vi "臂环接收机.vi"() -> ()   [LabVIEW 2023]
uses:
  <vilib>/Instr/_visa.llb/VISA Flush IO Buffer Mask.ctl
  <vilib>/Instr/_visa.llb/VISA Configure Serial Port (Instr).vi
panel:
  out "chn1":i32(graph)
  out "gry":cluster{i16, i16, i16}(graph)
  out "acc":cluster{i16, i16, i16}(graph)
  out "chn6":i32(graph)
  out "chn5":i32(graph)
  out "chn2":i32(graph)
  out "chn8":i32(graph)
  out "chn4":i32(graph)
  out "chn7":i32(graph)
  out "chn3":i32(graph)
  in  "write_buffer":string
  in  "发送按钮":bool
  out "ReadBuffer":string
  out "读取返回数":u32
  in  "serial":refnum<visa-resource-name> caption="VISA资源名称"
  in  "串口开关":bool
  out "串口状态":bool
  # "念通智能臂环软件——测试阶段试用版本"
  # "臂环通道1波形"
  # "臂环通道5波形"
  # "臂环通道2波形"
  # "臂环通道6波形"
  # "臂环通道3波形"
  # "臂环通道7波形"
  # "臂环通道4波形"
  # "臂环通道8波形"
  # "臂环角速度"
  # "臂环加速度表"
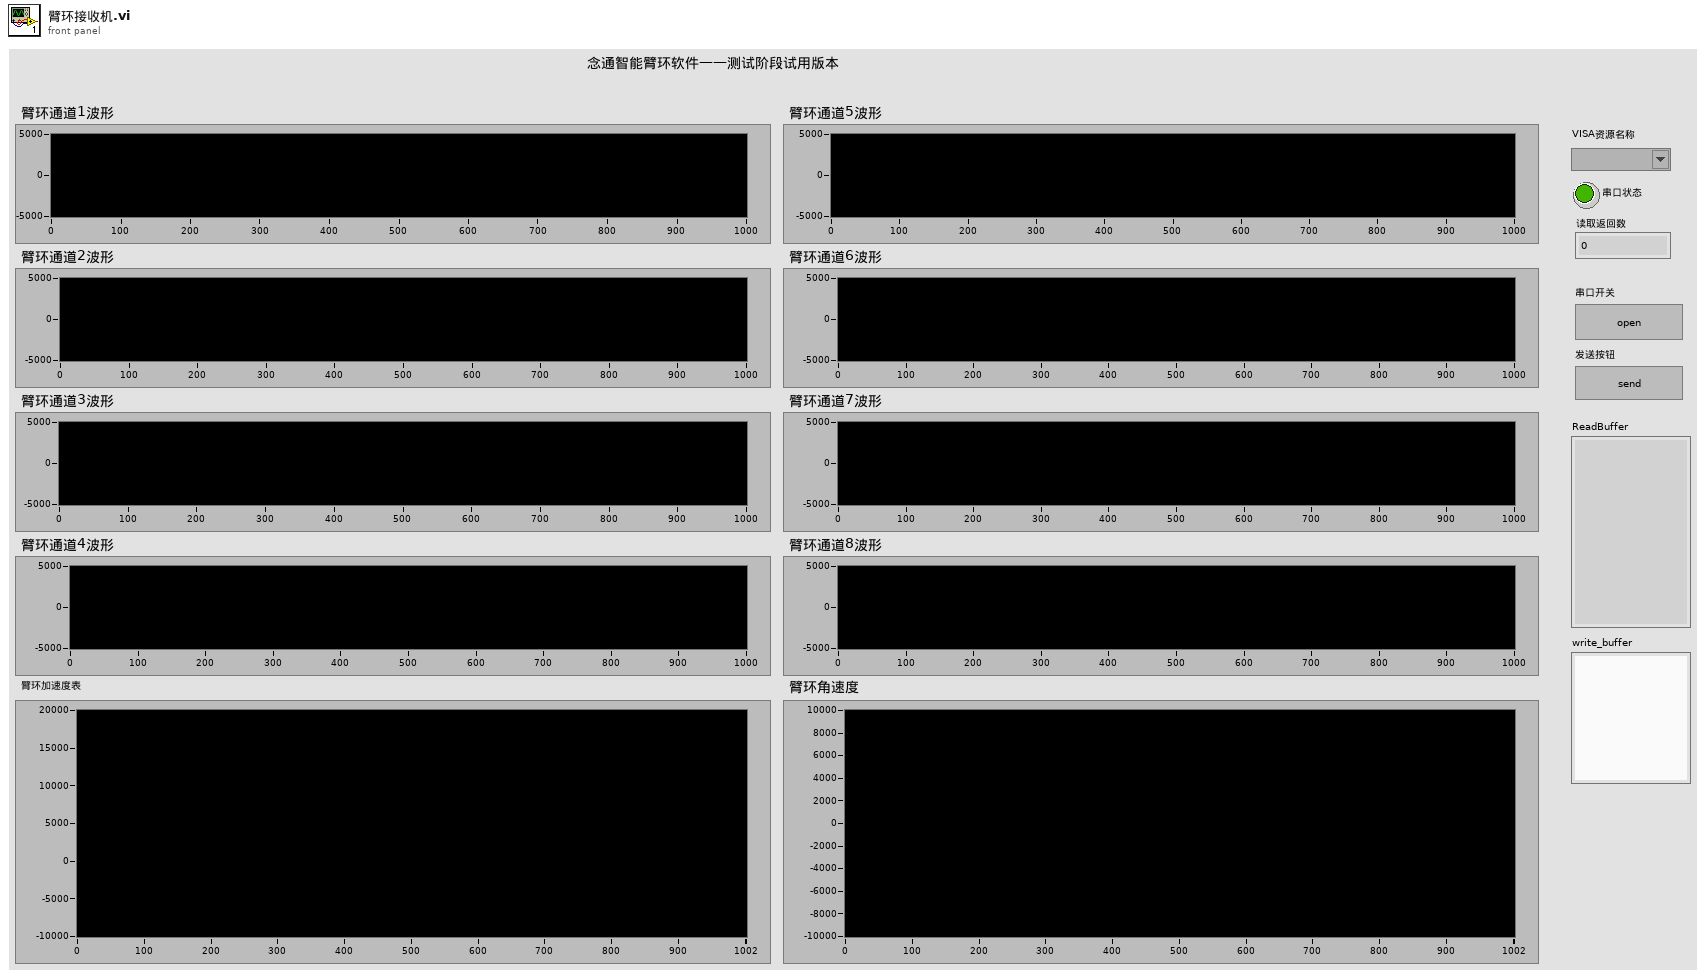
[diagram p1: front panel]
types:
  T1 = enum16{"nohead", "get_bb", "get_aa", "none_4bytes", "get_crc", "get_bat", "get_cnt"}
  T2 = cluster{"rx_cnt":u32, "rx_finish":bool, "head":enum16{"nohead", "get_bb", "get_aa", "none_4bytes", "get_crc", "get_bat", "get_cnt"}, "rx_len":u32, "data_len":u32, "crc":u8, "bat_lev":u8, "data":u8[], "none_4byte":u8[], "rx_4byte_len":u8}
  T3 = typedef "状态机控件.ctl" = enum16{"init_state", "main_state", "uart_receive_state", "stop_state"}
  T4 = typedef "VISA Flush IO Buffer Mask.ctl" = u16
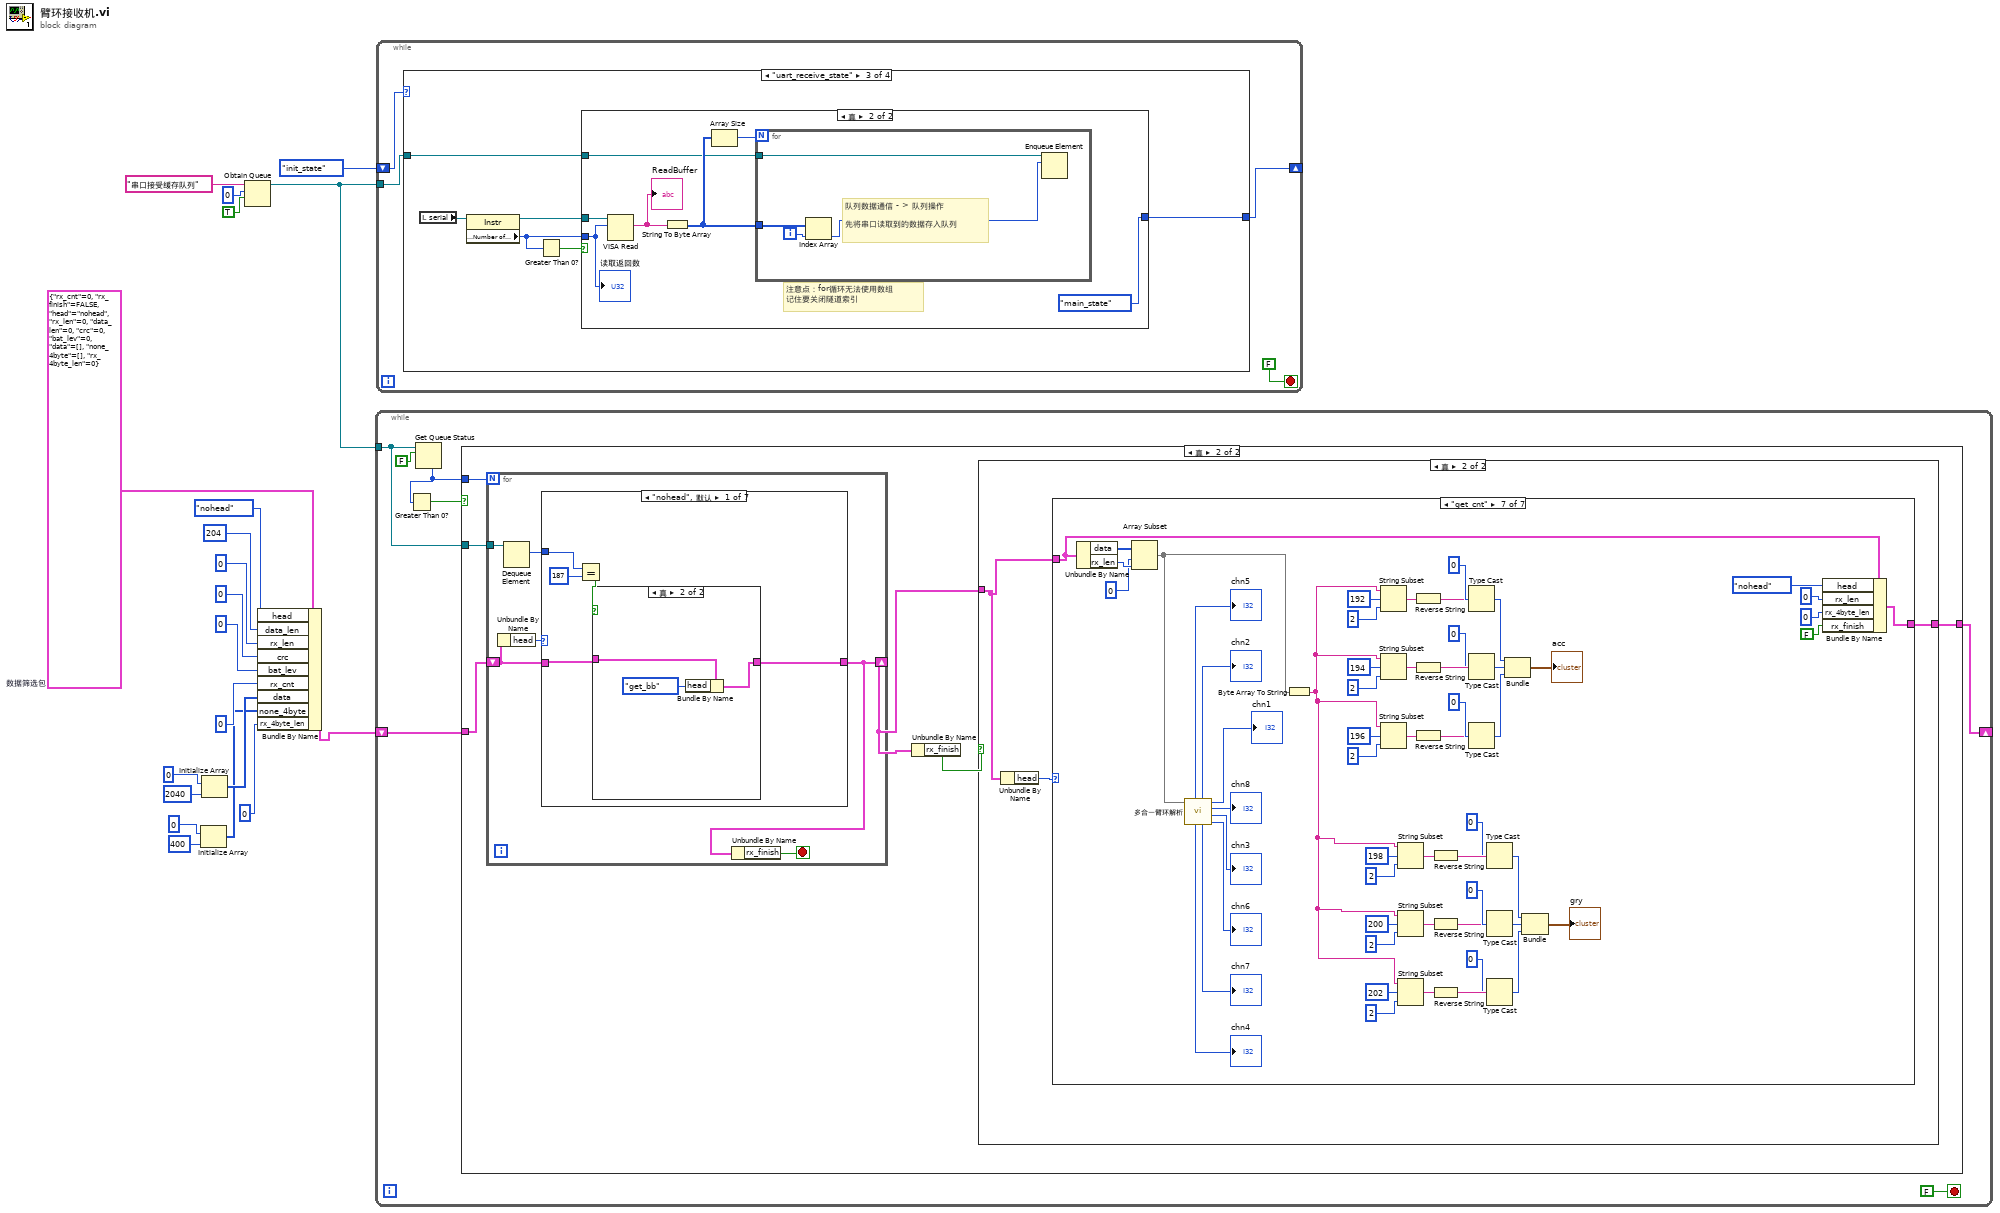
[diagram p0: block diagram]
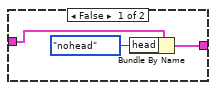
[diagram p10: hidden frame]
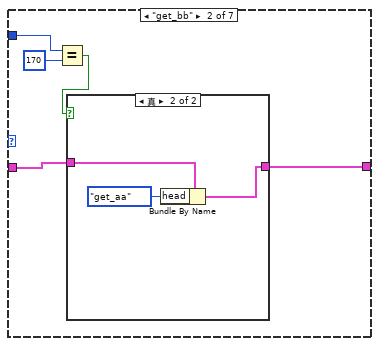
[diagram p11: hidden frame]
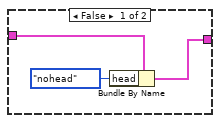
[diagram p12: hidden frame]
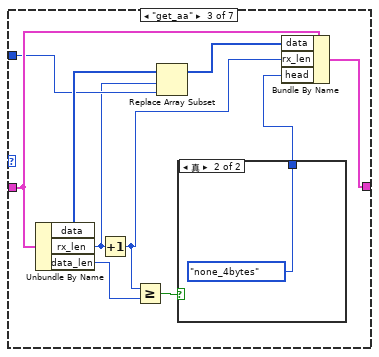
[diagram p13: hidden frame]
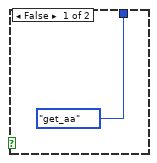
[diagram p14: hidden frame]
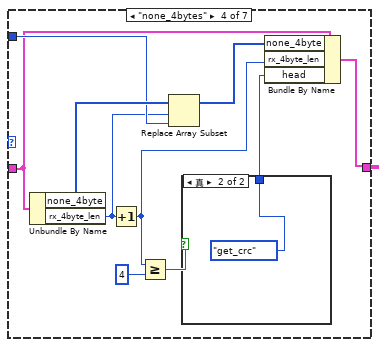
[diagram p15: hidden frame]
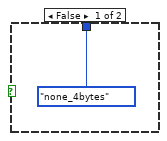
[diagram p16: hidden frame]
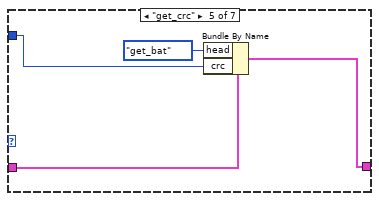
[diagram p17: hidden frame]
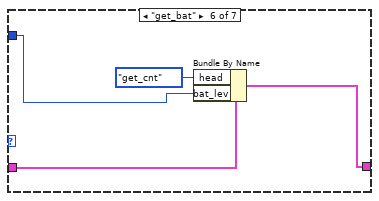
[diagram p18: hidden frame]
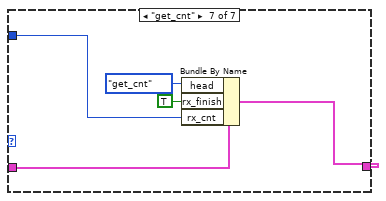
[diagram p19: hidden frame]
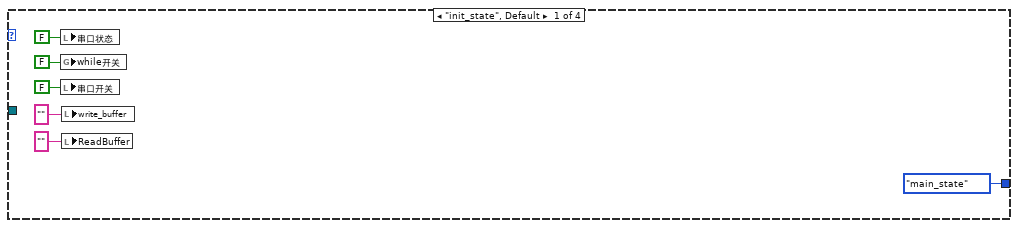
[diagram p20: hidden frame]
diagram:
  w2 = T2 {"rx_cnt"=0, "rx_finish"=FALSE, "head"=enum."nohead", "rx_len"=0, "data_len"=0, "crc"=0, "bat_lev"=0, "data"=[], "none_4byte"=[], "rx_4byte_len"=0}  # 数据筛选包
  n1 = Initialize Array(u8 0 ("元素"), 400 ("维数大小")) -> (w5:u8[])
  n2 = Initialize Array(u8 0 ("元素"), 2040 ("维数大小")) -> (w10:u8[])
  n3 = Obtain Queue(name (unnamed)="串口接受缓存队列" ("名称（未命名）"), element data type=u8 0, create if not found? (T)=TRUE ("如未找到则创建？(T)")) -> (queue out=w16:refnum<queue>)  [unwired: 2 in, 2 out]
  n4 = Bundle By Name(cluster=w2, "head"=T1."nohead", "data_len"=204, "rx_len"=0, "crc"=0, "bat_lev"=0, "rx_cnt"=u32 0, "data"=w10, "none_4byte"=w5, "rx_4byte_len"=u8 0) -> (w1:T2)
  n5 = while {
    tunnel: w16 -> [w22]
    shift-right: [w21] -> _
    shift-left: w1 -> [w23]
    stop <- FALSE stop-if-true
    n6 = Get Queue Status(queue=w22, return elements? (F)=FALSE ("返回元素？(F)")) -> (# elements in queue=w24:i32)  [unwired: 1 in, 7 out]
    n7 = Greater Than 0?(x=w24) -> (x > 0?=w25:bool)
    n8 = case shown="真" w25 {
      tunnel: w24 -> [_ w34]
      tunnel: w23 -> [w28 w33]
      tunnel: w22 -> [_ w32]
      tunnel: [w28 w29] -> w21
      frame False {
      }
      frame True {
        n9 = for {
          N: w34 -> [_]
          tunnel: w32 -> [w107]
          shift-right: [w103] -> w30
          shift-left: w33 -> [w104]
          stop <- w102 stop-if-true
          n10 = Unbundle By Name(w104) -> ("head"=w106:T1)
          n11 = Dequeue Element(queue=w107) -> (element=w105:u8)  [unwired: 2 in, 3 out]
          n12 = case shown="\"nohead\", 默认" w106 {
            tunnel: w105 -> [w111 w122 w135 w148 w155 w159 w165]
            tunnel: w104 -> [w109 w120 w139 w146 w157 w161 w166]
            tunnel: [w108 w119 w130 w142 w154 w158 w162] -> w103
            frame "nohead", Default {
              n13 = Equal?(x=w111, y=u8 187) -> (x = y?=w110:bool)
              n14 = case shown="真" w110 {
                tunnel: w109 -> [w115 w118]
                tunnel: [w113 w117] -> w108
                frame False {
                  n15 = Bundle By Name(cluster=w115, "head"=T1."nohead") -> (w113:T2)
                }
                frame True {
                  n16 = Bundle By Name(cluster=w118, "head"=T1."get_bb") -> (w117:T2)
                }
              }
            }
            frame "get_bb" {
              n17 = Equal?(x=w122, y=u8 170) -> (x = y?=w121:bool)
              n18 = case shown="真" w121 {
                tunnel: w120 -> [w125 w128]
                tunnel: [w124 w127] -> w119
                frame False {
                  n19 = Bundle By Name(cluster=w125, "head"=T1."nohead") -> (w124:T2)
                }
                frame True {
                  n20 = Bundle By Name(cluster=w128, "head"=T1."get_aa") -> (w127:T2)
                }
              }
            }
            frame "get_aa" {
              n21 = Unbundle By Name(w139) -> ("data"=w136:u8[], "rx_len"=w134:u32, "data_len"=w138:u32)
              n22 = Increment(x=w134) -> (x+1=w133:u32)
              n23 = Greater Or Equal?(x=w133, y=w138) -> (x >= y?=w137:bool)
              n24 = Replace Array Subset(array=w136, new element=w135, index=w134) -> (w132:u8[])
              n25 = case shown="真" w137 {
                tunnel: [T1."get_aa" ("head") T1."none_4bytes" ("head")] -> w131
                frame False {
                }
                frame True {
                }
              }
              n26 = Bundle By Name(cluster=w139, "data"=w132, "rx_len"=w133, "head"=w131) -> (w130:T2)
            }
            frame "none_4bytes" {
              n27 = Unbundle By Name(w146) -> ("none_4byte"=w149:u8[], "rx_4byte_len"=w147:u8)
              n28 = Increment(x=w147) -> (x+1=w144:u8)
              n29 = Greater Or Equal?(x=w144, y=u8 4) -> (x >= y?=w151:bool)
              n30 = Replace Array Subset(array=w149, new element=w148, index=w147) -> (w145:u8[])
              n31 = case shown="真" w151 {
                tunnel: [T1."none_4bytes" ("head") T1."get_crc" ("head")] -> w143
                frame False {
                }
                frame True {
                }
              }
              n32 = Bundle By Name(cluster=w146, "none_4byte"=w145, "rx_4byte_len"=w144, "head"=w143) -> (w142:T2)
            }
            frame "get_crc" {
              n33 = Bundle By Name(cluster=w157, "head"=T1."get_bat", "crc"=w155) -> (w154:T2)
            }
            frame "get_bat" {
              n34 = Bundle By Name(cluster=w161, "head"=T1."get_cnt", "bat_lev"=w159) -> (w158:T2)
            }
            frame "get_cnt" {
              n35 = Bundle By Name(cluster=w166, "head"=T1."get_cnt", "rx_finish"=TRUE, "rx_cnt"=w165) -> (w162:T2)
            }
          }
          n36 = Unbundle By Name(w103) -> ("rx_finish"=w102:bool)
        }
        n37 = Unbundle By Name(w30) -> ("rx_finish"=w31:bool)
        n38 = case shown="真" w31 {
          tunnel: w30 -> [w35 w37]
          tunnel: [w35 w36] -> w29
          frame False {
          }
          frame True {
            n39 = Unbundle By Name(w37) -> ("head"=w38:T1)
            n40 = case shown="\"get_cnt\"" w38 {
              tunnel: w37 -> [w39 w40 w41 w42 w43 w44 w98]
              tunnel: [w39 w40 w41 w42 w43 w44 w93] -> w36
              frame "nohead", Default {
              }
              frame "get_bb" {
              }
              frame "get_aa" {
              }
              frame "none_4bytes" {
              }
              frame "get_crc" {
              }
              frame "get_bat" {
              }
              frame "get_cnt" {
                n41 = Unbundle By Name(w98) -> ("data"=w101:u8[], "rx_len"=w100:u32)
                n42 = Array Subset(array=w101, index=u32 0 ("索引"), length=w100) -> (w85:u8[])
                n43 = call "多合一臂环解析.vi"("数组"=w85) -> ("chn6"=→"chn6":i32, "chn3"=→"chn3":i32, "chn8"=→"chn8":i32, "chn1"=→"chn1":i32, "chn7"=→"chn7":i32, "chn2"=→"chn2":i32, "chn4"=→"chn4":i32, "chn5"=→"chn5":i32)  [unwired: 3 in]
                n44 = Byte Array To String(unsigned byte array=w85) -> (string=w46:string)
                n45 = String Subset(string=w46, offset (0)=192 ("偏移量(0)"), length (rest)=2 ("长度（剩余）")) -> (substring=w82:string)
                n46 = String Subset(string=w46, offset (0)=194 ("偏移量(0)"), length (rest)=2 ("长度（剩余）")) -> (substring=w76:string)
                n47 = String Subset(string=w46, offset (0)=196 ("偏移量(0)"), length (rest)=2 ("长度（剩余）")) -> (substring=w71:string)
                n48 = String Subset(string=w46, offset (0)=198 ("偏移量(0)"), length (rest)=2 ("长度（剩余）")) -> (substring=w49:string)
                n49 = String Subset(string=w46, offset (0)=200 ("偏移量(0)"), length (rest)=2 ("长度（剩余）")) -> (substring=w55:string)
                n50 = String Subset(string=w46, offset (0)=202 ("偏移量(0)"), length (rest)=2 ("长度（剩余）")) -> (substring=w60:string)
                n51 = Reverse String(1:w82) -> (0:w80:string)
                n52 = Reverse String(1:w76) -> (0:w78:string)
                n53 = Reverse String(1:w71) -> (0:w69:string)
                n54 = Reverse String(1:w49) -> (0:w51:string)
                n55 = Reverse String(1:w55) -> (0:w53:string)
                n56 = Reverse String(1:w60) -> (0:w62:string)
                n57 = Type Cast(type=i16 0, x=w80) -> (*(type *) &x=w79:i16)
                n58 = Type Cast(type=i16 0, x=w78) -> (*(type *) &x=w68:i16)
                n59 = Type Cast(type=i16 0, x=w69) -> (*(type *) &x=w67:i16)
                n60 = Type Cast(type=i16 0, x=w51) -> (*(type *) &x=w52:i16)
                n61 = Type Cast(type=i16 0, x=w53) -> (*(type *) &x=w63:i16)
                n62 = Type Cast(type=i16 0, x=w62) -> (*(type *) &x=w64:i16)
                n63 = Bundle(w79, w68, w67) -> (→"acc":cluster{i16, i16, i16})  [unwired: 1 in]
                n64 = Bundle(w52, w63, w64) -> (→"gry":cluster{i16, i16, i16})  [unwired: 1 in]
                n65 = Bundle By Name(cluster=w98, "head"=T1."nohead", "rx_len"=u8 0, "rx_4byte_len"=u8 0, "rx_finish"=FALSE) -> (w93:T2)
              }
            }
          }
        }
      }
    }
  }
  n66 = while {
    shift-right: [w170] -> _
    shift-left: 状态机控件."init_state" ("枚举") -> [w169]
    tunnel: w16 -> [w168]
    stop <- FALSE stop-if-true
    n67 = case shown="\"uart_receive_state\"" w169 {
      tunnel: [状态机控件."main_state" ("枚举") w178 w213 状态机控件."stop_state" ("枚举")] -> w170
      tunnel: w168 -> [_ _ w208 _]
      frame "init_state", Default {
        n68 = local write "串口状态"(FALSE ("串口状态")) -> ()
        n69 = global write "枚举全局变量.vi" "while开关"(FALSE ("全局变量while开关")) -> ()
        n70 = local write "串口开关"(FALSE ("串口状态")) -> ()
        n71 = local write "write_buffer"("" ("write_buffer")) -> ()
        n72 = local write "ReadBuffer"("" ("ReadBuffer")) -> ()
      }
      frame "main_state" {
        n73 = event shown="[1] \"串口开关\": 值改变" {
          selector: _ -> [_ _ _]
          dyn-events: _ -> [_ _ _]
          timeout: 0 -> [_ _ _]
          tunnel: [w180 w183 w201] -> w178
          event Timeout {
            n74 = event-data() -> ()  [unwired: 1 in, 3 out]
            n75 = local read "串口状态"() -> (w179:bool)
            n76 = case shown="假" w179 {
              tunnel: [状态机控件."main_state" ("枚举") 状态机控件."uart_receive_state" ("枚举")] -> w180
              frame False {
              }
              frame True {
              }
            }
          }
          event "串口开关": Value Change {
            n77 = event-data() -> ()  [unwired: 1 in, 6 out]
            n78 = case shown="假" "串口开关" {
              tunnel: [状态机控件."main_state" ("枚举") w188] -> w183
              frame False {
                # "关闭串口"
                n79 = local read "serial"() -> (w186:refnum<visa-resource-name>)
                n80 = local write "串口状态"(FALSE ("串口状态")) -> ()
                n81 = VISA Close(VISA resource name=w186) -> ()  [unwired: 1 in, 1 out]
              }
              frame True {
                n82 = call-poly "VISA Configure Serial Port"("VISA resource name"="serial", "baud rate (9600)"=u32 921600) -> ("error out"=w191:errorcluster)  [unwired: 12 in, 1 out]
                n83 = Unbundle By Name(w191) -> ("status"=w190:bool)
                n84 = Not(x=w190) -> (.not. x?=w189:bool)
                "串口状态" <- w189
                n85 = case shown="真" w189 {
                  tunnel: [状态机控件."main_state" ("枚举") 状态机控件."uart_receive_state" ("枚举")] -> w188
                  frame False {
                    n86 = local write "串口开关"(FALSE ("串口状态")) -> ()
                    n87 = One Button Dialog(message="串口打开失败" ("消息")) -> ()  [unwired: 1 in, 1 out]
                  }
                  frame True {
                    w197 = T4 16 items=["清空接收缓冲区"=16, "向设备写入传输缓冲区"=32, "清空接收缓冲区（无I/O）"=64, "清空传输缓冲区"=128] ("Mask")
                    n88 = local read "serial"() -> (w198:refnum<visa-resource-name>)
                    n89 = VISA Flush I/O Buffer(VISA resource name=w198, mask (16)=w197) -> ()  [unwired: 1 in, 2 out]
                  }
                }
              }
            }
          }
          event "发送按钮": Value Change {
            n90 = event-data() -> ()  [unwired: 1 in, 6 out]
            n91 = local read "串口状态"() -> (w200:bool)
            n92 = case shown="真" w200 {
              tunnel: [状态机控件."main_state" ("枚举") 状态机控件."uart_receive_state" ("枚举")] -> w201
              frame False {
                n93 = One Button Dialog(message="打开串口后在发送" ("消息")) -> ()  [unwired: 1 in, 1 out]
              }
              frame True {
                n94 = global write "枚举全局变量.vi" "while开关"(FALSE ("while开关")) -> ()
                n95 = local read "serial"() -> (w207:refnum<visa-resource-name>)
                n96 = VISA Write(VISA resource name=w207, write buffer="write_buffer") -> ()  [unwired: 1 in, 3 out]
              }
            }
          }
        }
      }
      frame "uart_receive_state" {
        n97 = local read "serial"() -> (w209:refnum<visa-resource-name>)
        n98 = property class="Instr"(reference=w209) -> (reference out=w211:refnum<visa-resource-name>, "Serial Settings:Number of Bytes at Serial Port"=w210:u32)  [unwired: 1 in, 1 out]
        n99 = Greater Than 0?(x=w210) -> (x > 0?=w212:bool)
        n100 = case shown="真" w212 {
          tunnel: [状态机控件."main_state" ("枚举") 状态机控件."main_state" ("枚举")] -> w213
          tunnel: w211 -> [_ w220]
          tunnel: w210 -> [_ w219]
          tunnel: w208 -> [_ w215]
          frame False {
          }
          frame True {
            # "注意点：for循环无法使用数组\n记住要关闭隧道索引"
            n101 = VISA Read(VISA resource name=w220, byte count=w219) -> (read buffer=w218:string)  [unwired: 1 in, 3 out]
            "ReadBuffer" <- w218
            n102 = String To Byte Array(string=w218) -> (unsigned byte array=w216:u8[])
            n103 = Array Size(array=w216) -> (size(s)=w217:i32)
            n104 = for {
              N: w217 -> [_]
              tunnel: w216 -> [w225]
              tunnel: w215 -> [w223]
              i -> [w224]
              # "队列数据通信 - > 队列操作\n\n先将串口读取到的数据存入队列"
              n105 = Index Array(array=w225, index=w224) -> (element=w222:u8)
              n106 = Enqueue Element(queue=w223, element=w222) -> ()  [unwired: 2 in, 3 out]
            }
            "读取返回数" <- w219
          }
        }
      }
      frame "stop_state" {
      }
    }
  }
